vi "SelectGroup.vi"(8 "error in (no error)":errorcluster, 11 "ClassDataTree in":refnum<class "ClassDataTree.lvclass">) -> (0 "error out":errorcluster, 3 "ClassDataTree out":refnum<class "ClassDataTree.lvclass">)   [LabVIEW 2016, in "ClassDataTree.lvclass"]
uses:
  ClassDataTree.lvclass
  ClassDataTree.lvclass/ClassDataTree.ctl
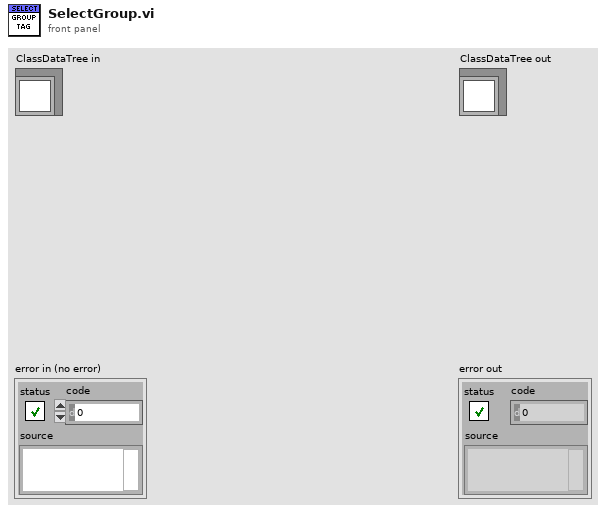
[diagram p1: front panel]
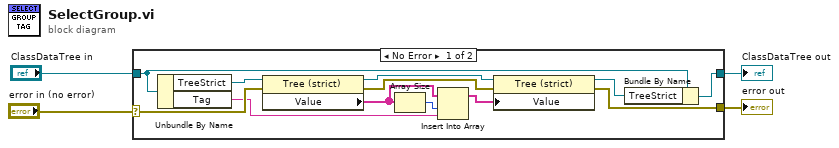
[diagram p0: block diagram]
diagram:
  n1 = case shown="No Error" "error in (no error)" {
    selector: "error in (no error)" -> [w10 w18]
    tunnel: [w8 w18] -> w3
    tunnel: [w11 w17] -> w1
    tunnel: "ClassDataTree in" -> [w13 w17]
    frame No Error {
      n2 = Unbundle By Name(w13) -> ("TreeStrict"=w14:refnum<vi>, "Tag"=w7:string)
      n3 = property class="Tree (strict)"(reference=w14, error in=w10) -> (reference out=w15:refnum<vi>, error out=w9:errorcluster, "Value"=w6:string[])
      n4 = Array Size(array=w6) -> (size(s)=w5:i32)
      n5 = Insert Into Array(array=w6, index=w5, new element=w7) -> (w16:string[])
      n6 = property class="Tree (strict)"(reference=w15, error in=w9, "Value"=w16) -> (reference out=w12:refnum<vi>, error out=w8:errorcluster)
      n7 = Bundle By Name(cluster=w13, "TreeStrict"=w12) -> (w11:refnum<class "ClassDataTree.lvclass">)
    }
    frame Error {
    }
  }
  "error out" <- w3
  "ClassDataTree out" <- w1
